vi "Sensor Interface View.vi"(8 "error in (no error)":errorcluster, 11 "View Model":T1) -> (0 "error out":errorcluster, 3 "View Model":T1)   [LabVIEW 2013]
doc: "Simulates the elevator position transducer/switch."
uses:
  View Model/Controls/View Model.ctl
  Error/Controls/Error Model.ctl
  Error/Controls/Error Types.ctl
  View Model/Controls/Shared Model.ctl
  Elevator Controller/Controls/Elevator Model.ctl
  Elevator Controller/Controls/Controller Overhead.ctl
  Elevator Controller/Controls/Elevator States.ctl
  Elevator Controller/Controls/Elevator Location.ctl
  Elevator Controller/Controls/Elevator Command Event.ctl
  Elevator Controller/Controls/Elevator Commands.ctl
  Configuration/Controls/Configuration Model.ctl
  Configuration/Controls/Configuration Data.ctl
panel:
  out "Elevator Position":u16(slide)=1 min=1 max=4 step=1 scale=1.0..4.0
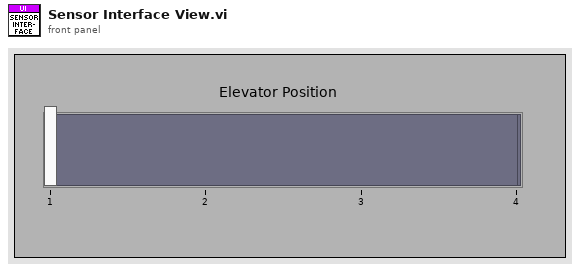
[diagram p1: front panel]
types:
  T1 = typedef "View Model.ctl" = cluster{"Error Model":T2, "Shared Model":T3, "Elevator Model":T4, "Configuration Model":T5}
  T2 = typedef "Error Model.ctl" = cluster{"Error Event":refnum<user-event>}
  T3 = typedef "Shared Model.ctl" = cluster{"Stop DVR":refnum<data-value>, "Stop Event":refnum<user-event>}
  T4 = typedef "Elevator Model.ctl" = cluster{"Controller Overhead":refnum<data-value>, "Motion Change":refnum<user-event>, "Direction Change":refnum<user-event>, "Door Position Change":refnum<user-event>, "Emergency Change":refnum<user-event>, "Floor Change":refnum<user-event>, "Elevator Cmd":refnum<user-event>}
  T5 = typedef "Configuration Model.ctl" = cluster{"Configuration":refnum<data-value>, "Config Change":refnum<user-event>}
  T6 = typedef "Elevator Location.ctl" = enum16{"1st Floor", "2nd Floor", "3rd Floor", "4th Floor"}
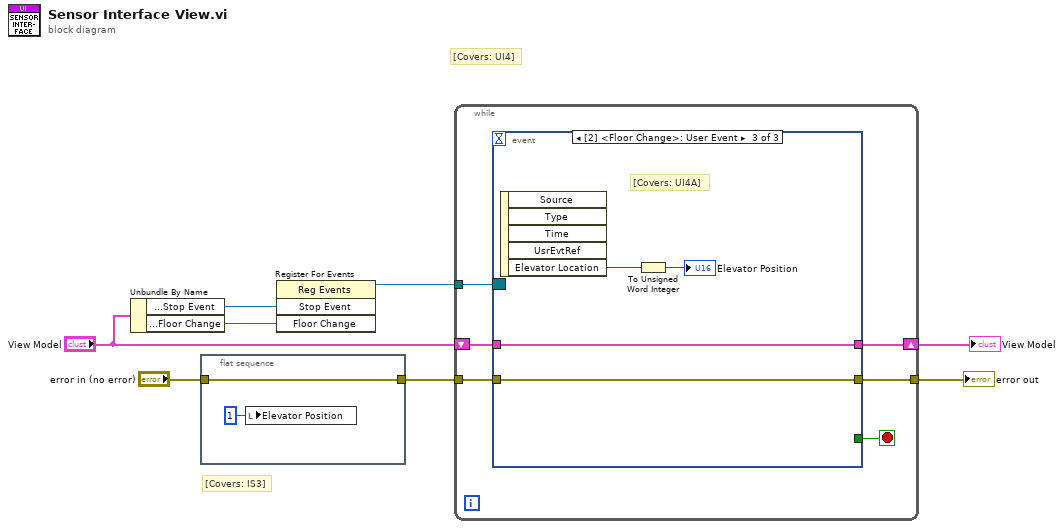
[diagram p0: block diagram]
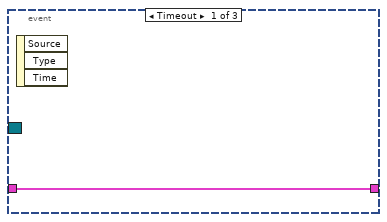
[diagram p2: hidden frame]
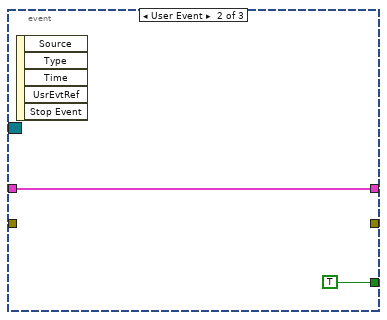
[diagram p3: hidden frame]
diagram:
  # "[Covers: UI4]"
  # "[Covers: IS3]"
  n1 = Unbundle By Name("View Model") -> ("Shared Model.Stop Event"=w8:refnum<user-event>, "Elevator Model.Floor Change"=w5:refnum<user-event>)
  n2 = flat-sequence {
    tunnel: "error in (no error)" -> [w9]
    tunnel: [w9] -> w1
    frame #0 {
      n3 = local write "Elevator Position"(u16 1 ("Elevator Position")) -> ()
    }
  }
  n4 = register-events(w8, w5) -> (reference out=w7:refnum<event-registration>)  [unwired: 2 in, 1 out]
  n5 = while {
    tunnel: w7 -> [w16]
    tunnel: w1 -> [w13]
    shift-right: [w12] -> w4
    shift-left: "View Model" -> [w14]
    tunnel: [w11] -> w3
    stop <- w15 stop-if-true
    n6 = event shown="[2] <Floor Change>: User Event" {
      selector: w16 -> [_ _ _]
      dyn-events: _ -> [_ _ _]
      timeout: _ -> [_ _ _]
      tunnel: [_ TRUE _] -> w15
      tunnel: w14 -> [w17 w18 w21]
      tunnel: w13 -> [_ _ w20]
      tunnel: [w17 w18 w21] -> w12
      tunnel: [_ _ w20] -> w11
      event Timeout {
        n7 = event-data() -> ()  [unwired: 1 in, 3 out]
      }
      event User Event {
        n8 = event-data() -> ()  [unwired: 1 in, 5 out]
      }
      event User Event {
        # "[Covers: UI4A]"
        n9 = event-data() -> ("Elevator Location"=w23:T6)  [unwired: 1 in, 4 out]
        n10 = To Unsigned Word Integer(number=w23) -> (unsigned 16bit integer=→"Elevator Position":u16)
      }
    }
  }
  "error out" <- w3
  "View Model" <- w4
